vi "NI VeriStand - Set FIFO Depth.vi"(8 "error in (no error)":errorcluster, 9 "Size FIFO Sink (1)":u32=1, 10 "Size FIFO Source (1)":u32=1, 11 "Device Ref in":T1 format="%.0x") -> (0 "error out":errorcluster, 3 "Device Ref out":T1 format="%.0x")   [LabVIEW 2020, in "Custom Device API.lvlib"]
doc: "Sets the depths of FIFOs for a custom device. NI VeriStand uses the FIFOs to share data with the RT engine. Use this VI only in a custom device RT VI that you launch asynchronously."
uses:
  <vilib>/NI VeriStand/Custom Device API/Custom Device API.lvlib
  <vilib>/NI VeriStand/Custom Device API/Custom Device Item Ref.ctl
  29a590d7-8992-4b63-a353-7bd8bf641803.vi
  <vilib>/NI VeriStand/Custom Device API/Custom Device Offline Path.vi
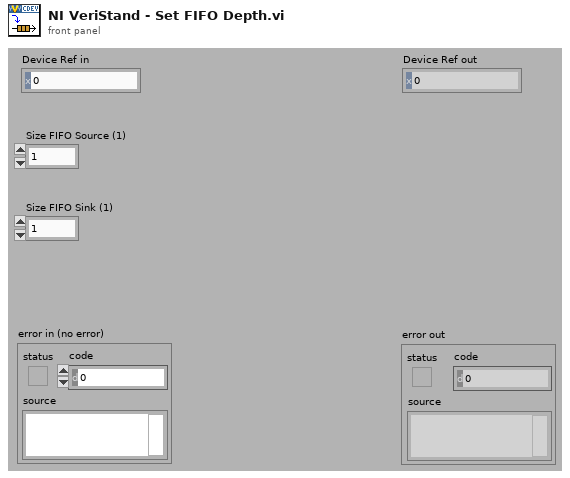
[diagram p1: front panel]
types:
  T1 = typedef "Custom Device API.lvlib/Custom Device Item Ref.ctl" = u64
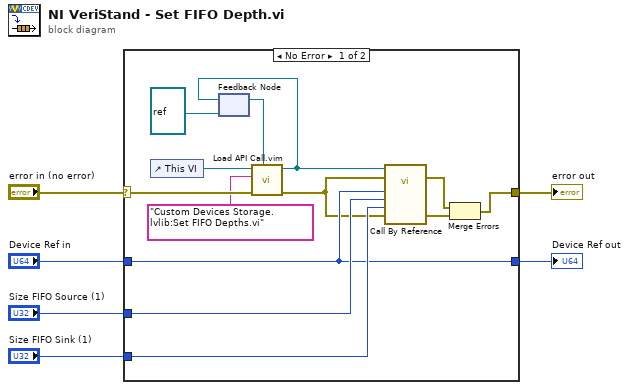
[diagram p0: block diagram]
diagram:
  n1 = case shown="No Error" "error in (no error)" {
    selector: "error in (no error)" -> [w12 w21]
    tunnel: [w18 w21] -> w6
    tunnel: "Device Ref in" -> [w15 w20]
    tunnel: "Size FIFO Source (1)" -> [w17 _]
    tunnel: "Size FIFO Sink (1)" -> [w16 _]
    tunnel: [w15 w20] -> w2
    frame No Error {
      n2 = control-ref of="This VI"() -> (w13:refnum<vi>)
      n3 = feedback #1(refnum<vi> refnum ("type specifier VI Refnum (for type only)")) -> (w14:refnum<vi>)
      n4 = call "Load API Call.vim"("VI reference in"=w14, "error in (no error)"=w12, "VI qualified name"="Custom Devices Storage.lvlib:Set FIFO Depths.vi", "Caller VI ref"=w13) -> ("error out"=w11:errorcluster, "VI reference"=w10:refnum<vi>)  [unwired: 6 in]
      n5 = feedback-in #1(w10) -> ()
      n6 = call-by-ref "?"(reference=w10, error in=w11, 8:"error in (no error)"=w11, "Size FIFO Sink (1)"=w16, "Size FIFO Source (1)"=w17, "Device Ref in"=w15) -> (error out=w7:errorcluster, 0:"error out"=w19:errorcluster)  [unwired: 6 in, 2 out]
      n7 = Merge Errors(w7, w19) -> (w18:errorcluster)
    }
    frame Error {
    }
  }
  "Device Ref out" <- w2
  "error out" <- w6
